vi "Greatest Common Prime Factor (GCPF)-array input.vi"(8 "error in (no error)":errorcluster) -> (0 "error out":errorcluster, 2 "T = the input integers are relatively prime":bool, 3 "Greatest Common Prime Factor (GCPF)":i32)   [LabVIEW 2021, in "Numeric Utilities.lvlib"]
uses:
  Numeric Utilities.lvlib
  Factors cluster.ctl
panel:
  out "Dev: List of factors (ascending length)":T1[][](array[typedef])
  out "Dev: Factor list lengths":i32[](array[numeric])
  in  "Integers":i32[](array[numeric])
  out "Dev: prime divisors common to all input integers":i32[](array[numeric])
  # "Development\ncontrols/indicators useful for development and testing, but which are not outputs of the VI"
  # "Input\nInputs to the VI"
  # "Output\nOutputs of the VI"
  # "Description\n\nBlank VI with error handling case. \n\nSummarize the use of this VI in this space."
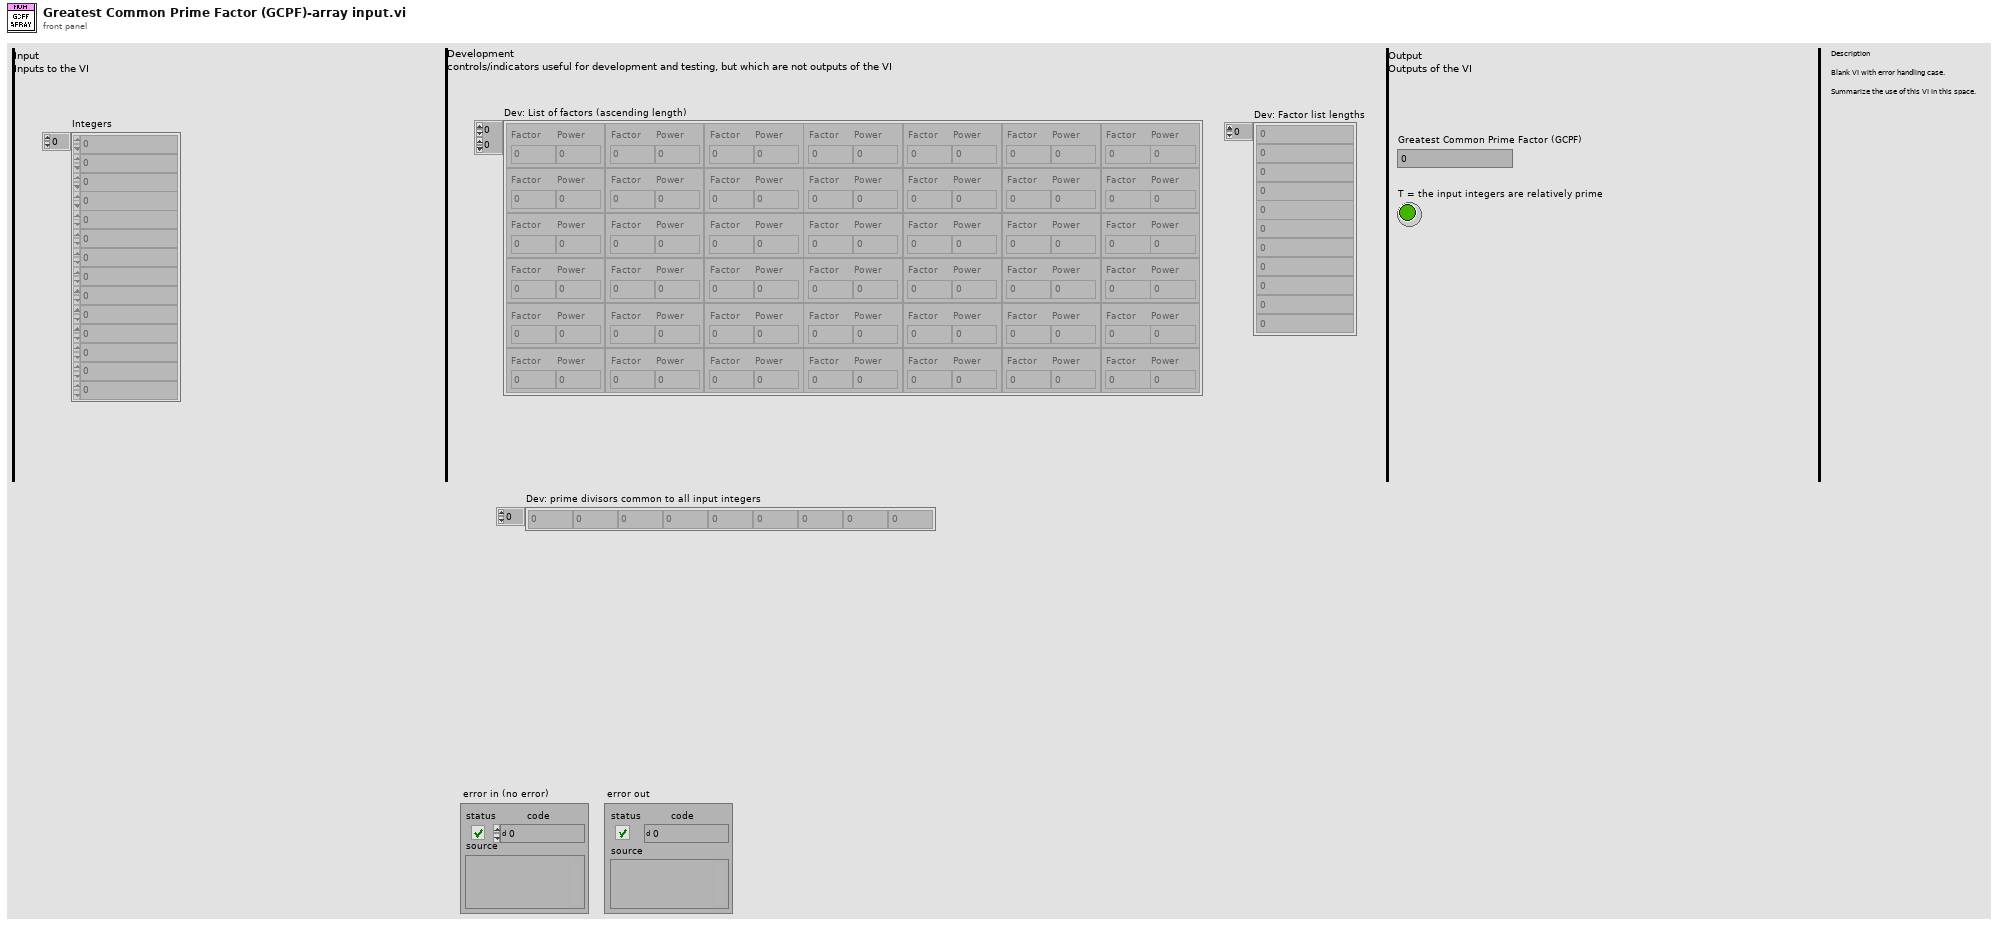
[diagram p1: front panel]
types:
  T1 = typedef "Numeric Utilities.lvlib/Factors cluster.ctl" = cluster{"Factor":i32, "Power":i32}
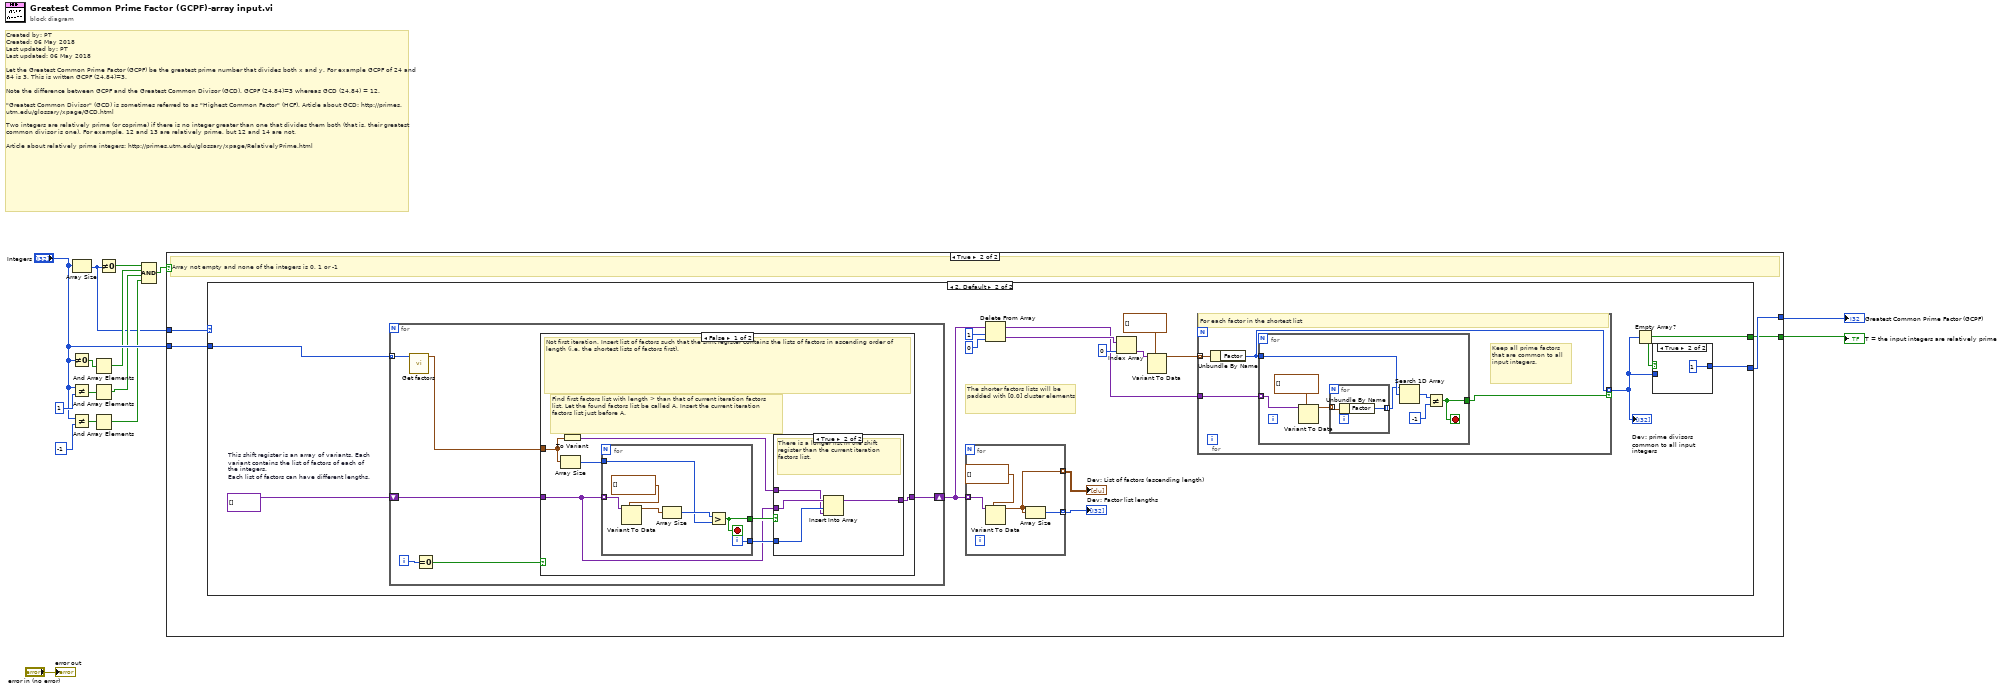
[diagram p0: block diagram]
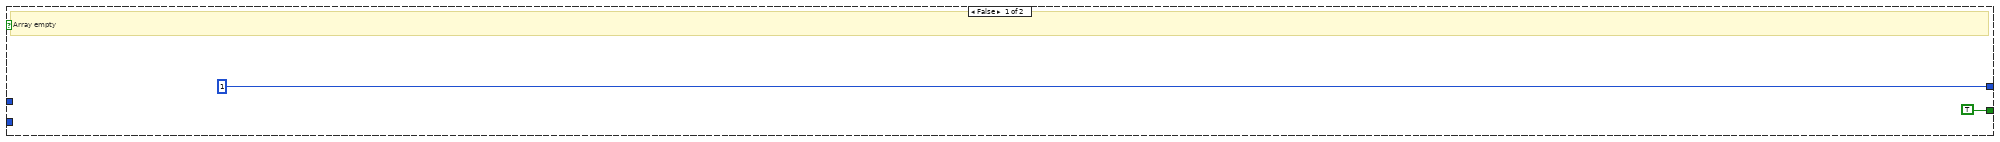
[diagram p2: hidden frame]
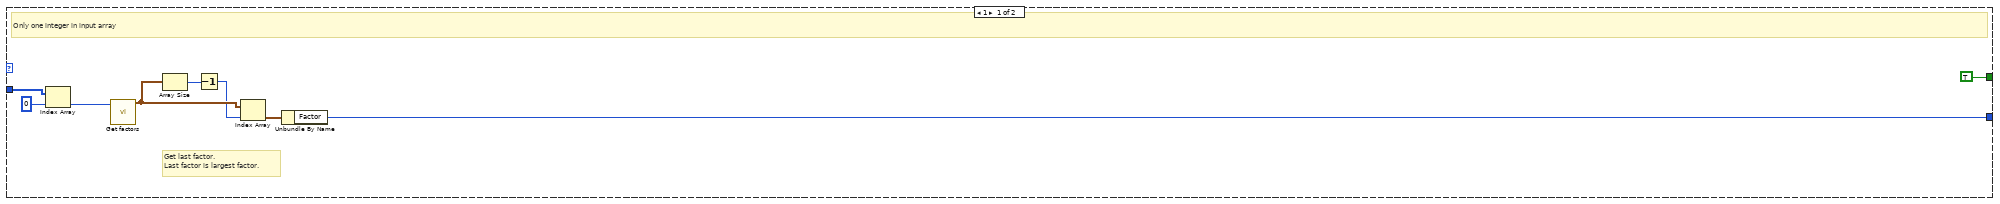
[diagram p3: hidden frame]
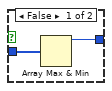
[diagram p4: hidden frame]
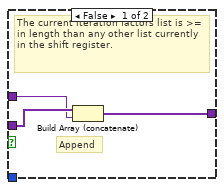
[diagram p5: hidden frame]
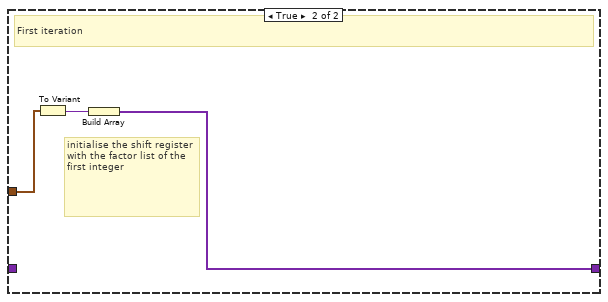
[diagram p6: hidden frame]
diagram:
  # "Created by: PT\nCreated: 06 May 2018\nLast updated by: PT\nLast updated: 06 May 2018\n\nLet the Greatest Common Prime Factor (GCPF) be the greatest prime number that divides both x and y. For example GCPF of 24 and 84 is 3. This is written GCPF (24,84)=3.\n\nNote the difference between GCPF and the Greatest Common Divisor (GCD). GCPF (24,84)=3 whereas GCD (24,84) = 12.\n\n\"Greatest Common Divisor\" (GCD) is sometimes referred to as \"Highest Common Factor\" (HCF). Article about GCD: http://primes.utm.edu/glossary/xpage/GCD.html\n\nTwo integers are relatively prime (or coprime) if there is no integer greater than one that divides them both (that is, their greatest common divisor is one). For example, 12 and 13 are relatively prime, but 12 and 14 are not.\n\nArticle about relatively prime integers: http://primes.utm.edu/glossary/xpage/RelativelyPrime.html"
  n1 = Array Size(array="Integers") -> (size(s)=w2:i32)
  n2 = Not Equal To 0?(x="Integers") -> (x != 0?=w14:bool[])
  n3 = Not Equal?(x="Integers", y=1) -> (x != y?=w12:bool[])
  n4 = Not Equal?(x="Integers", y=-1) -> (x != y?=w10:bool[])
  n5 = And Array Elements(Boolean array=w14) -> (logical AND=w7:bool)
  n6 = And Array Elements(Boolean array=w12) -> (logical AND=w6:bool)
  n7 = And Array Elements(Boolean array=w10) -> (logical AND=w5:bool)
  n8 = Not Equal To 0?(x=w2) -> (x != 0?=w3:bool)
  n9 = Compound Arithmetic op=AND(w3, w7, w6, w5) -> (w8:bool)
  n10 = case shown="True" w8 {
    tunnel: [1 w19] -> w4
    tunnel: "Integers" -> [_ w21]
    tunnel: w2 -> [_ w20]
    tunnel: [TRUE ("empty?") w18] -> w1
    frame False {
      # "Array empty"
    }
    frame True {
      # "Array not empty and none of the integers is 0, 1 or -1"
      n11 = case shown="2, Default" w20 {
        tunnel: w21 -> [w30 w46]
        tunnel: [w23 w35] -> w19
        tunnel: [TRUE ("empty?") w31] -> w18
        frame 1 {
          # "Get last factor.\nLast factor is largest factor."
          # "Only one integer in input array"
          n12 = Index Array(array=w30, index=0) -> (element=w28:i32)
          n13 = call "Get factors.vi"("x"=w28) -> ("Factors out"=w26:T1[])  [unwired: 5 in, 5 out]
          n14 = Array Size(array=w26) -> (size(s)=w27:i32)
          n15 = Decrement(x=w27) -> (x-1=w25:i32)
          n16 = Index Array(array=w26, index=w25) -> (element=w24:T1)
          n17 = Unbundle By Name(w24) -> ("Factor"=w23:i32)
        }
        frame 2, Default {
          w45 = variant[] []  # This shift register is an array of variants. Each variant contains the list of factors of each of the integers. Each list of factors can have different lengths.
          # "The shorter factors lists will be padded with [0,0] cluster elements"
          n18 = for {
            tunnel: w46 -> [w73] mode=indexing
            shift-right: [w69] -> w44
            shift-left: w45 -> [w68]
            i -> [w72]
            n19 = call "Get factors.vi"("x"=w73) -> ("Factors out"=w70:T1[])  [unwired: 5 in, 5 out]
            n20 = Equal To 0?(x=w72) -> (x = 0?=w71:bool)
            n21 = case shown="False" w71 {
              tunnel: w70 -> [w77 w97]
              tunnel: [w74 w95] -> w69
              tunnel: w68 -> [w75 _]
              frame False {
                # "Find first factors list with length > than that of current iteration factors list. Let the found factors list be called A. Insert the current iteration factors list just before A."
                # "Not first iteration. Insert list of factors such that the shift register contains the lists of factors in ascending order of length (i.e. the shortest lists of factors first)."
                n22 = Array Size(array=w77) -> (size(s)=w80:i32)
                n23 = To Variant(anything=w77) -> (Variant=w76:variant)
                n24 = for {
                  tunnel: w75 -> [w94] mode=indexing
                  tunnel: w80 -> [w90]
                  tunnel: [w89] -> w79
                  tunnel: [w88] -> w78
                  i -> [w88]
                  stop <- w89 stop-if-true
                  n25 = Variant To Data(type=T1[] [] ("Factors out"), Variant=w94) -> (data=w92:T1[])  [unwired: 1 in, 1 out]
                  n26 = Array Size(array=w92) -> (size(s)=w91:i32)
                  n27 = Greater?(x=w91, y=w90) -> (0:w89:bool)
                }
                n28 = case shown="True" w79 {
                  tunnel: w78 -> [_ w86]
                  tunnel: w76 -> [w82 w85]
                  tunnel: w75 -> [w83 w87]
                  tunnel: [w81 w84] -> w74
                  frame False {
                    # "Append"
                    # "The current iteration factors list is >= in length than any other list currently in the shift register."
                    n29 = Build Array (concatenate)(w83, w82) -> (w81:variant[])
                  }
                  frame True {
                    # "There is a longer list in the shift register than the current iteration factors list."
                    n30 = Insert Into Array(array=w87, index=w86, new element=w85) -> (w84:variant[])
                  }
                }
              }
              frame True {
                # "initialise the shift register with the factor list of the first integer"
                # "First iteration"
                n31 = To Variant(anything=w97) -> (Variant=w96:variant)
                n32 = Build Array(w96) -> (w95:variant[])
              }
            }
          }
          n33 = for {
            tunnel: w44 -> [w67] mode=indexing
            tunnel: [w65] -> w33 mode=indexing
            tunnel: [w64] -> w34 mode=indexing
            n34 = Variant To Data(type=T1[] [] ("Factors out"), Variant=w67) -> (data=w64:T1[])  [unwired: 1 in, 1 out]
            n35 = Array Size(array=w64) -> (size(s)=w65:i32)
          }
          "Dev: Factor list lengths" <- w33
          "Dev: List of factors (ascending length)" <- w34
          n36 = Delete From Array(array=w44, length=1, index=0) -> (deleted portion=w41:variant[], array with subset deleted=w36:variant[])
          n37 = Index Array(array=w41, index=0) -> (element=w39:variant)
          n38 = Variant To Data(type=T1[] [] ("Factors out"), Variant=w39) -> (data=w37:T1[])  [unwired: 1 in, 1 out]
          n39 = for {
            tunnel: w37 -> [w52] mode=indexing
            tunnel: w36 -> [w53]
            tunnel: [w50] -> w32 mode=indexing if=w51
            # "Keep all prime factors that are common to all input integers."
            # "For each factor in the shortest list"
            n40 = Unbundle By Name(w52) -> ("Factor"=w50:i32)
            n41 = for {
              tunnel: w50 -> [w59]
              tunnel: w53 -> [w60] mode=indexing
              tunnel: [w56] -> w51
              stop <- w56 stop-if-true
              n42 = Variant To Data(type=T1[] [] ("Factors out"), Variant=w60) -> (data=w55:T1[])  [unwired: 1 in, 1 out]
              n43 = for {
                tunnel: w55 -> [w63] mode=indexing
                tunnel: [w62] -> w54 mode=indexing
                n44 = Unbundle By Name(w63) -> ("Factor"=w62:i32)
              }
              n45 = Search 1D Array(1D array=w54, element=w59) -> (index of element=w58:i32)  [unwired: 1 in]
              n46 = Not Equal?(x=w58, y=-1) -> (x != y?=w56:bool)
            }
          }
          "Dev: prime divisors common to all input integers" <- w32
          n47 = Empty Array?(array=w32) -> (empty?=w31:bool)
          n48 = case shown="True" w31 {
            tunnel: [w48 1] -> w35
            tunnel: w32 -> [w47 _]
            frame False {
              n49 = Array Max & Min(array=w47) -> (max value=w48:i32)  [unwired: 3 out]
            }
            frame True {
            }
          }
        }
      }
    }
  }
  "T = the input integers are relatively prime" <- w1
  "Greatest Common Prime Factor (GCPF)" <- w4
  "error out" <- "error in (no error)"
